vi "FlagObjectArray_get_and_lock.vi"(8 "error in (no error)":errorcluster) -> (0 "error out":errorcluster, 3 "FlagObjects":refnum<class "flag.lvclass">[](array[class]))   [LabVIEW 2017]
doc: "the VI locks and returns/reads the FlagObjectsArray using a Queue"
uses:
  Classes/Flags/flag.lvclass
  global variables.vi
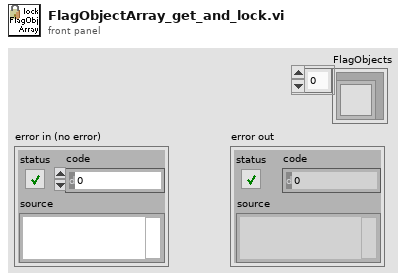
[diagram p1: front panel]
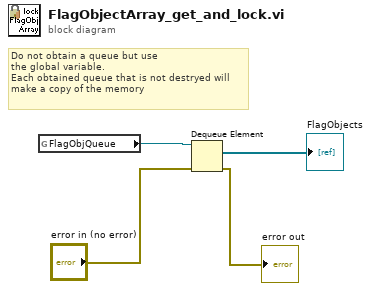
[diagram p0: block diagram]
diagram:
  # "Do not obtain a queue but use\nthe global variable.\nEach obtained queue that is not destryed will\nmake a copy of the memory"
  n1 = global read "global variables.vi" "FlagObjQueue"() -> (w3:refnum<queue>)
  n2 = Dequeue Element(queue=w3, error in (no error)="error in (no error)") -> (element=→"FlagObjects":refnum<class "flag.lvclass">[], error out=→"error out":errorcluster)  [unwired: 1 in, 2 out]
